vi "bubble sorting.vi"(10 "Array":dbl[](array[numeric])) -> (3 "sorted":dbl[](array[numeric]))   [LabVIEW 2014]
panel:
  out "Sorted Array":dbl[](array[numeric])
  out "swap":bool
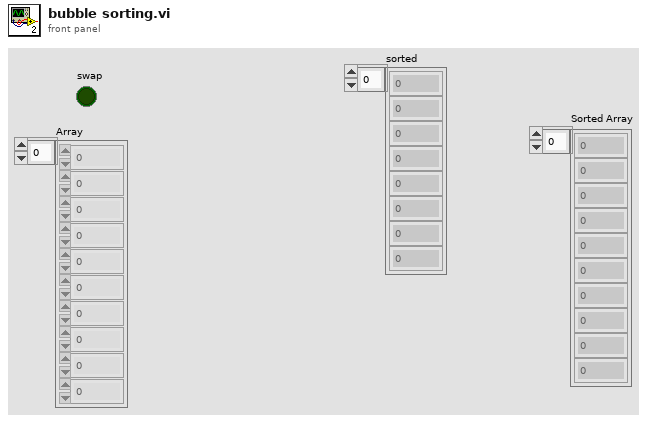
[diagram p1: front panel]
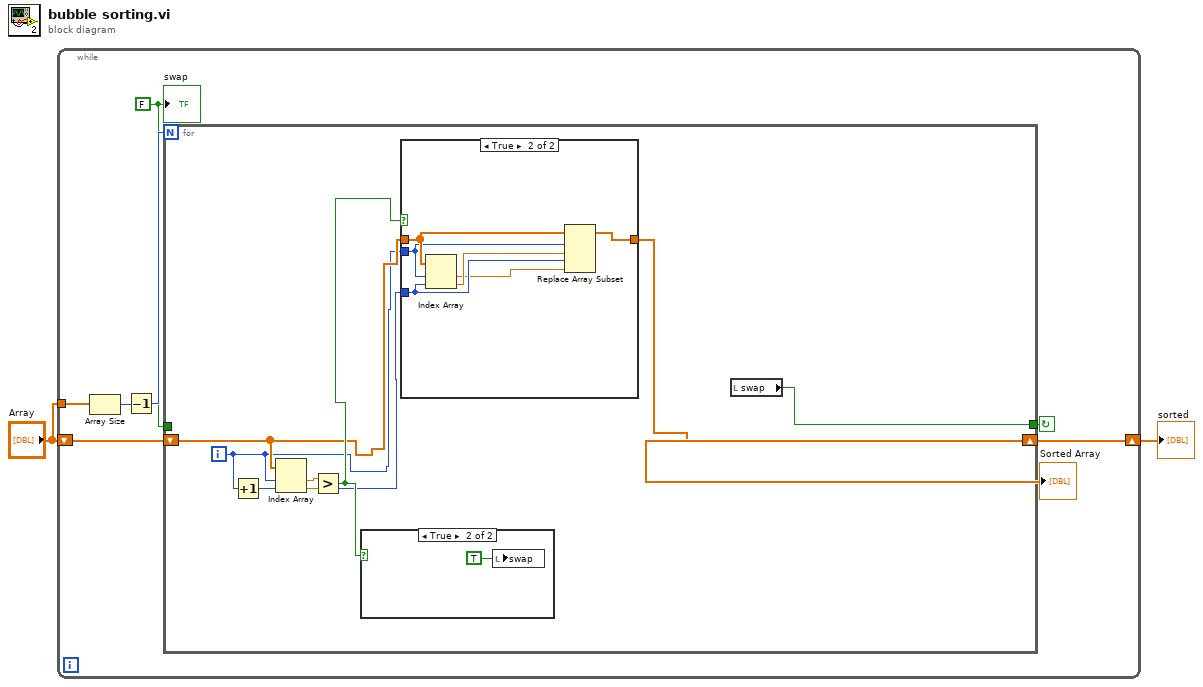
[diagram p0: block diagram]
diagram:
  n1 = while {
    tunnel: "Array" -> [w6]
    shift-right: [w3] -> w1
    shift-left: "Array" -> [w5]
    stop <- w4 continue-if-true
    w7 = FALSE
    n2 = Array Size(array=w6) -> (size(s)=w9:i32)
    n3 = Decrement(x=w9) -> (x-1=w8:i32)
    n4 = for {
      N: w8 -> [_]
      shift-right: [w10] -> w3
      shift-left: w5 -> [w13]
      tunnel: w7 -> [_]
      tunnel: [w15] -> w4
      i -> [w12]
      n5 = Increment(x=w12) -> (x+1=w11:i32)
      n6 = Index Array(array=w13, index #1=w12, index #2=w11) -> (element #1=w17:dbl, element #2=w16:dbl)
      n7 = Greater?(x=w17, y=w16) -> (0:w14:bool)
      n8 = case shown="True" w14 {
        frame False {
        }
        frame True {
          n9 = local write "swap"(TRUE) -> ()
        }
      }
      n10 = case shown="True" w14 {
        tunnel: w13 -> [w18 w24]
        tunnel: w12 -> [_ w23]
        tunnel: w11 -> [_ w21]
        tunnel: [w18 w19] -> w10
        frame False {
        }
        frame True {
          n11 = Index Array(array=w24, index #1=w23, index #2=w21) -> (element #1=w20:dbl, element #2=w22:dbl)
          n12 = Replace Array Subset(array=w24, new element #1=w22, index #1=w23, new element #2=w20, index #2=w21) -> (w19:dbl[])
        }
      }
      n13 = local read "swap"() -> (w15:bool)
    }
    "Sorted Array" <- w3
    "swap" <- w7
  }
  "sorted" <- w1
